vi "Add New to Project.vi"(8 "error in (no error)":errorcluster, 10 "Owning Library":refnum<vi>, 11 "Path":path) -> (0 "error out":errorcluster)   [LabVIEW 2020, in "Mock Class Updater.lvclass"]
uses:
  Mock Class Updater.lvclass
  Mock Class Updater.lvclass/Mock Class Updater.ctl
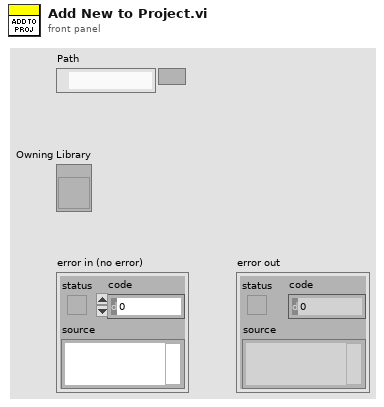
[diagram p1: front panel]
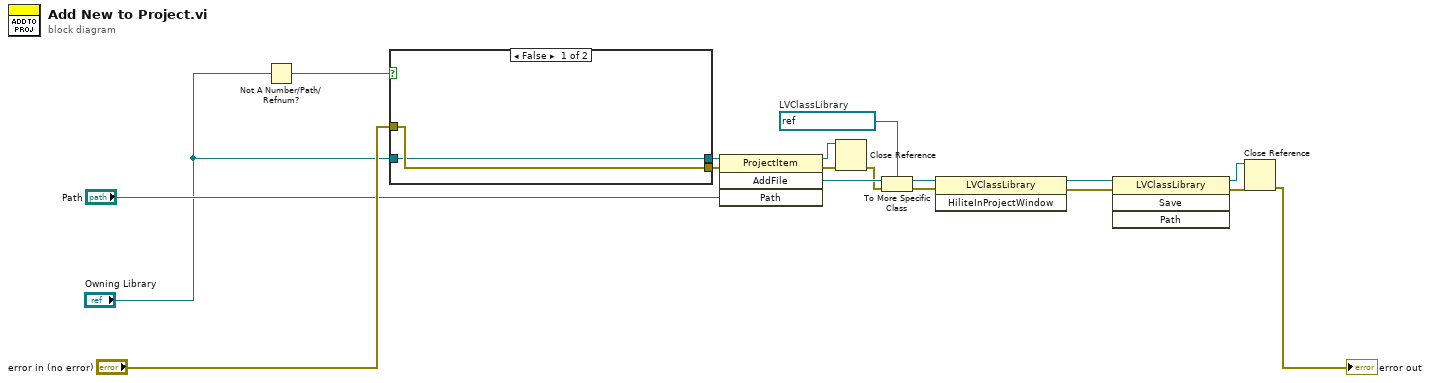
[diagram p0: block diagram]
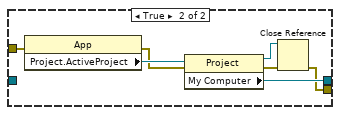
[diagram p2: hidden frame]
diagram:
  w13 = refnum<vi> refnum  # LVClassLibrary
  n1 = Not A Number/Path/Refnum?(number/path/refnum="Owning Library") -> (NaN/Path/Refnum?=w2:bool)
  n2 = case shown="False" w2 {
    tunnel: [w19 w26] -> w15
    tunnel: [w20 w22] -> w12
    tunnel: "error in (no error)" -> [w20 w21]
    tunnel: "Owning Library" -> [w19 _]
    frame False {
    }
    frame True {
      n3 = property class="App"(error in=w21) -> (error out=w25:errorcluster, "Project.ActiveProject"=w27:refnum<vi>)  [unwired: 1 in, 1 out]
      n4 = property class="Project"(reference=w27, error in=w25) -> (reference out=w23:refnum<vi>, error out=w24:errorcluster, "My Computer"=w26:refnum<vi>)
      n5 = Close Reference(reference=w23, error in (no error)=w24) -> (error out=w22:errorcluster)
    }
  }
  n6 = invoke class="ProjectItem" method="AddFile"(reference=w15, error in=w12, "Path"="Path") -> (reference out=w11:refnum<vi>, error out=w10:errorcluster, "AddFile"=w14:refnum<vi>)  [unwired: 1 in, 1 out]
  n7 = Close Reference(reference=w11, error in (no error)=w10) -> (error out=w9:errorcluster)
  n8 = To More Specific Class(target class=w13, reference=w14, error in=w9) -> (specific class reference=w7:refnum<vi>, error out=w5:errorcluster)
  n9 = invoke class="LVClassLibrary" method="HiliteInProjectWindow"(reference=w7, error in=w5) -> (reference out=w6:refnum<vi>, error out=w4:errorcluster)  [unwired: 1 in, 1 out]
  n10 = invoke class="LVClassLibrary" method="Save"(reference=w6, error in=w4) -> (reference out=w16:refnum<vi>, error out=w17:errorcluster)  [unwired: 2 in, 2 out]
  n11 = Close Reference(reference=w16, error in (no error)=w17) -> (error out=→"error out":errorcluster)
